vi "fit_c_axis.vi"(7 "Grain Number":i32, 8 "Error In":errorcluster, 10 "Sample":string, 11 "File Path Control":path) -> (0 "Error Out":errorcluster, 1 "Best R2":dbl, 2 "Phi min":dbl, 3 "Theta min":dbl)   [LabVIEW 2019]
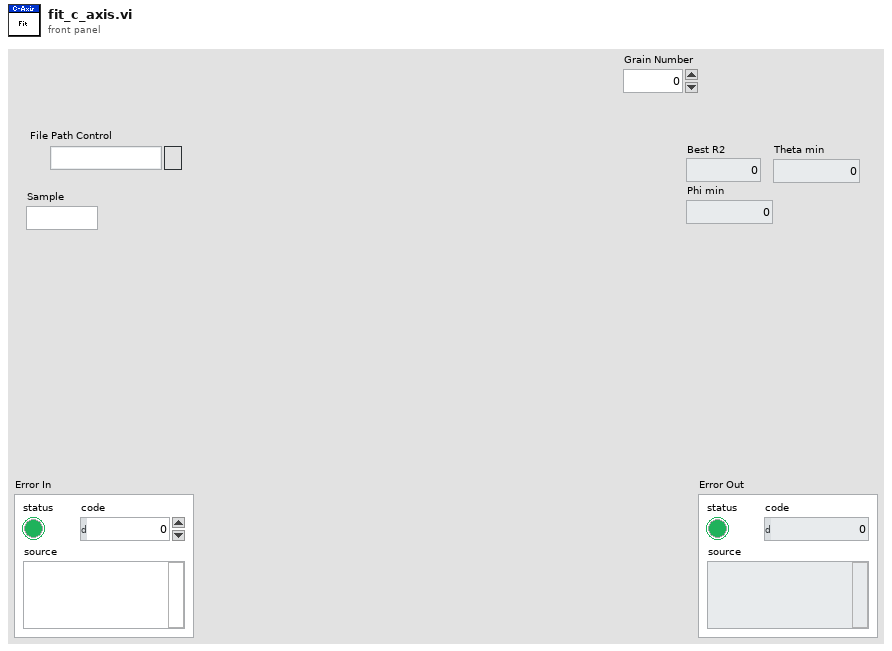
[diagram p1: front panel]
types:
  T1 = typedef "sample_results_cluster_typedef.ctl" = cluster{"File Path":string, "Sample":string, "Threshold":dbl, "Parameters":T2, "Writeable Parameters":T3, "Gain Results":T4[]}
  T2 = typedef "parameters_cluster_typedef.ctl" = cluster{"m1":dbl, "m2":dbl, "m3":dbl, "c":dbl, "D":dbl, "Beta":dbl, "center x":dbl, "center y":dbl}
  T3 = typedef "writeable_section_parameters_cluster_typedef.ctl" = cluster{"Section":string, "Method":i32, "Edge Mode":i32, "Grid Constant":i32, "Manual Sequence":i32, "ROI Size":i32, "Min Grain Size":dbl, "Comments":string, "File Path":string}
  T4 = typedef "grain_results_cluster_typedef.ctl" = cluster{"Grain Number":i32, "xi":dbl[], "phiin":dbl[], "Intensity":dbl[][], "Best Fit Intensity":dbl[][], "Best Fit Parameters":dbl[][], "Polarizer 1 Angle":dbl[][], "Polarizer 2 Angle":dbl[][], "Best Extinction Angle":dbl[], "Best Extinction Angle Corrected":dbl[], "Thetac":dbl, "Phic":dbl, "ROI":cluster{"Global Rectangle":i32[], "Contours":cluster{"Contour Type":u32, "ROI Type":u32, "Points":i32[]}[]}, "a":dbl, "b":dbl, "sequences available":dbl, "sequences used":dbl, "Contrast":dbl[], "Rsq":dbl}
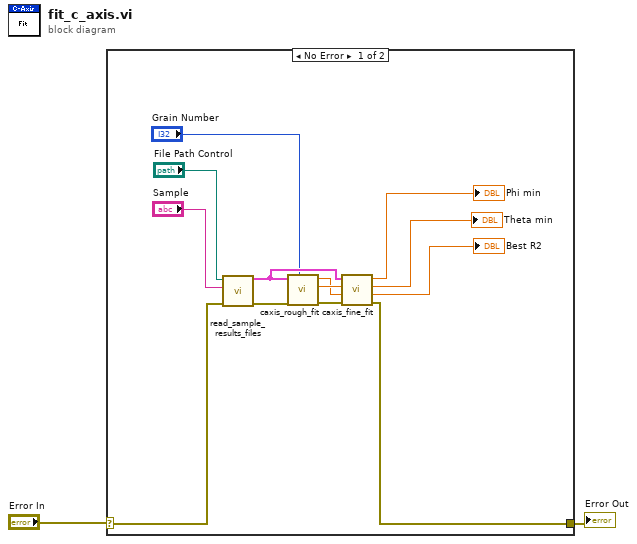
[diagram p0: block diagram]
diagram:
  n1 = case shown="No Error" "Error In" {
    selector: "Error In" -> [w13 w16]
    tunnel: [w4 w16] -> w1
    frame No Error {
      n2 = call "read_sample_results_files.vi"("Error In"=w13, "Sample"="Sample", "File Path"="File Path Control") -> ("Error Out"=w12:errorcluster, "Sample Results"=w10:T1)  [unwired: 7 in]
      n3 = call "caxis_rough_fit.vi"("Grain Number"="Grain Number", "Error In"=w12, "Sample Results"=w10) -> ("Error Out"=w11:errorcluster, "Theta min"=w9:dbl, "Phi min"=w8:dbl)  [unwired: 5 in, 1 out]
      n4 = call "caxis_fine_fit.vi"("Error In"=w11, "phic start"=w8, "thetac start"=w9, "Sample Results"=w10) -> ("Error Out"=w4:errorcluster, "Best R2"=→"Best R2":dbl, "Theta min"=→"Theta min":dbl, "Phi min"=→"Phi min":dbl)  [unwired: 4 in]
    }
    frame Error {
    }
  }
  "Error Out" <- w1
